vi "IB_RW_Project_Destination_Absolute.vi"(7 "action":T1, 8 "ErrIn":errorcluster, 9 "index":string, 10 "Path":path, 11 "buildObject":T2) -> (0 "ErrOut":errorcluster, 1 "index out":string, 2 "Path":path, 3 "buildObject out":T2)   [LabVIEW 2020]
uses:
  <resource>/Framework/Providers/API/ItemRef.ctl
  <vilib>/AppBuilder/IB_RW_Project/IB_RW_Project_PropBag_Action.ctl
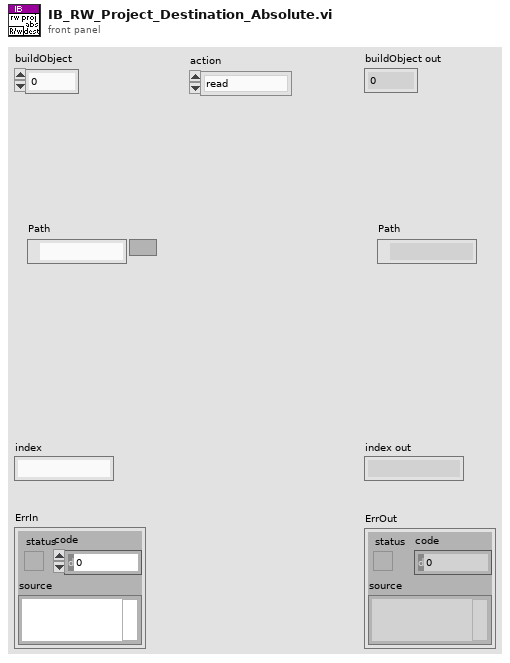
[diagram p1: front panel]
types:
  T1 = typedef "IB_RW_Project_PropBag_Action.ctl" = enum16{"read", "write", "clear", "readPrevious", "writePrevious", "clearPrevious"}
  T2 = typedef "ItemRef.ctl" = u64
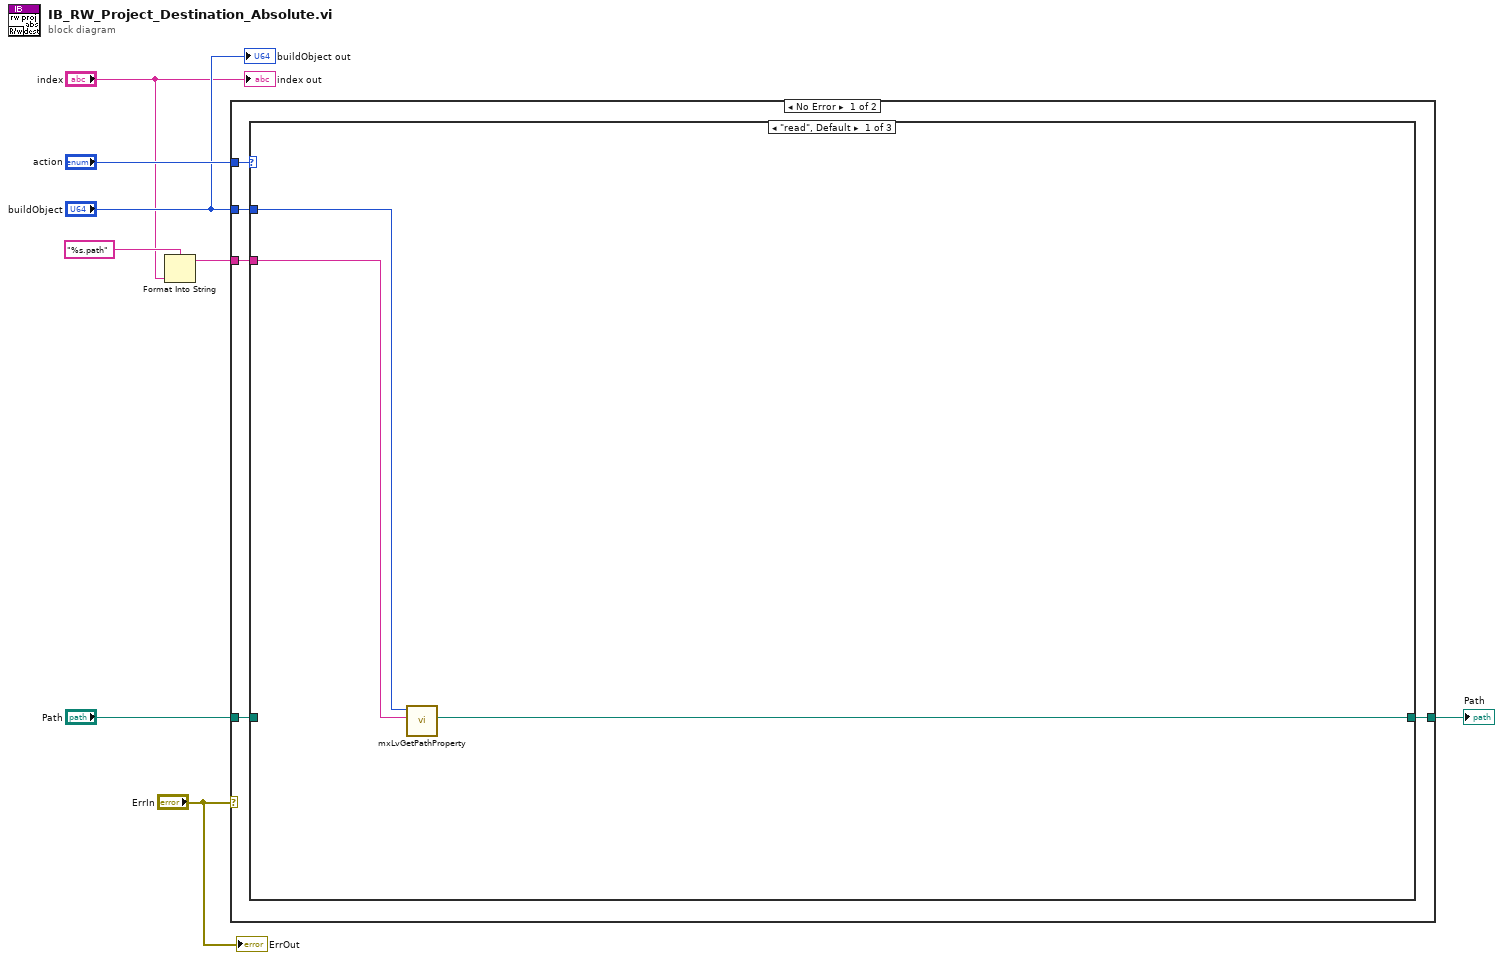
[diagram p0: block diagram]
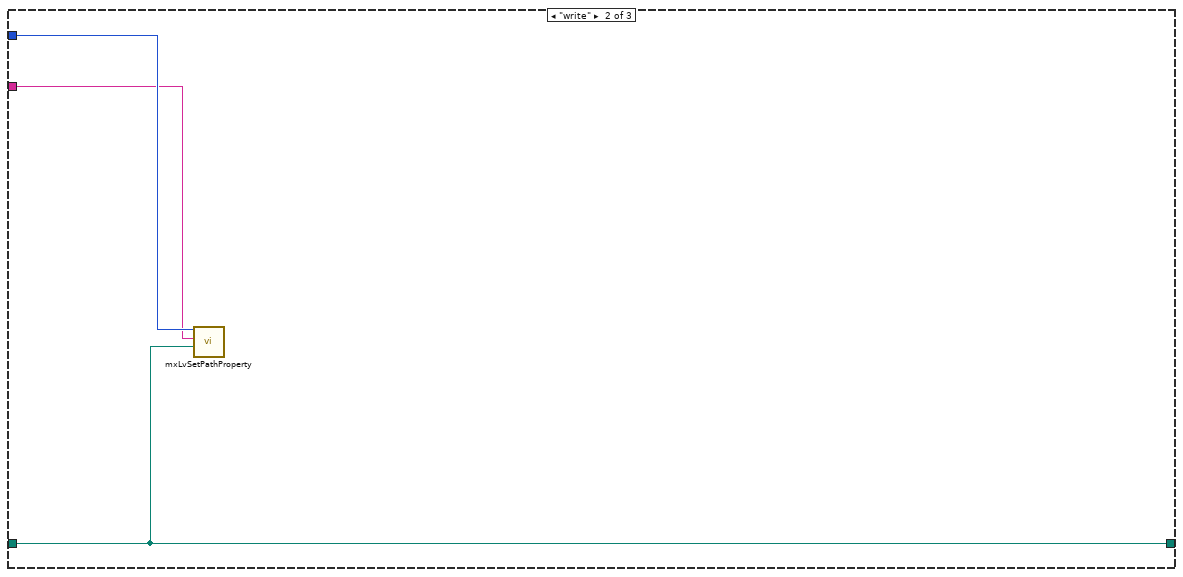
[diagram p2: hidden frame]
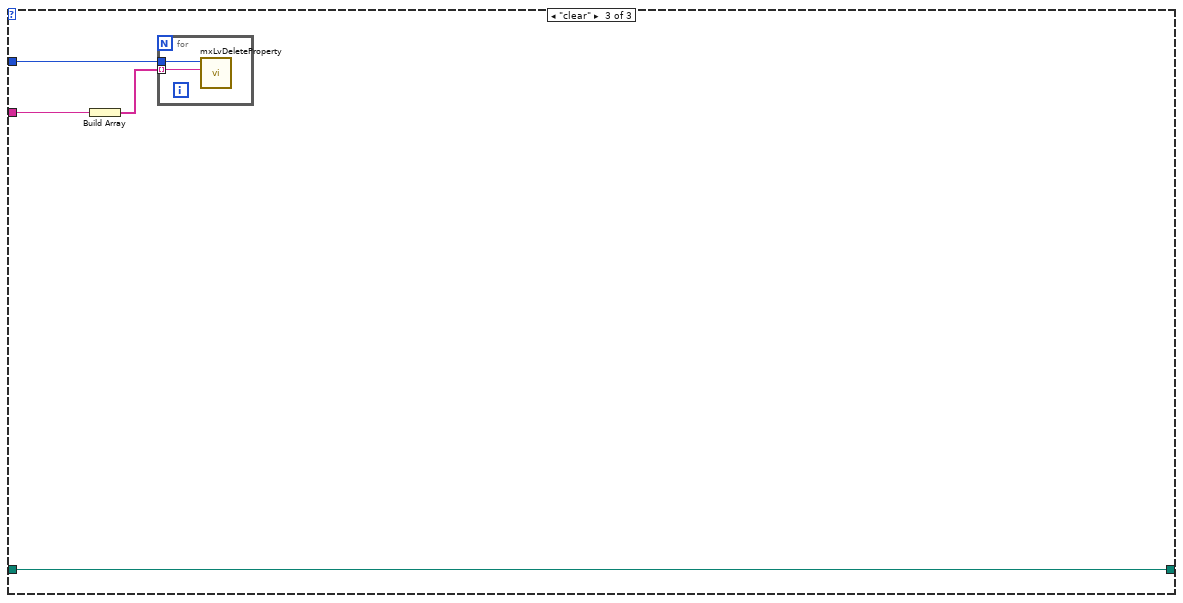
[diagram p3: hidden frame]
diagram:
  n1 = Format Into String(format string="%s.path", "index") -> (resulting string=w4:string)  [unwired: 2 in, 1 out]
  n2 = case shown="No Error" "ErrIn" {
    tunnel: "action" -> [w13 _]
    tunnel: "buildObject" -> [w12 _]
    tunnel: "Path" -> [w11 w26]
    tunnel: [w10 w26] -> w3
    tunnel: w4 -> [w9 _]
    frame No Error {
      n3 = case shown="\"read\", Default" w13 {
        tunnel: w12 -> [w16 w19 w23]
        tunnel: w11 -> [_ w17 w20]
        tunnel: [w14 w17 w20] -> w10
        tunnel: w9 -> [w15 w18 w22]
        frame "read", Default {
          n4 = call <resource>:"mxLvGetPathProperty.vi"("Tag"=w15, "Item"=w16) -> ("Path"=w14:path)  [unwired: 7 in, 2 out]
        }
        frame "write" {
          n5 = call <resource>:"mxLvSetPathProperty.vi"("Path"=w17, "Tag"=w18, "Item"=w19) -> ()  [unwired: 7 in, 2 out]
        }
        frame "clear" {
          n6 = Build Array(w22) -> (w21:string[])
          n7 = for {
            tunnel: w23 -> [w25]
            tunnel: w21 -> [w24] mode=indexing
            n8 = call <resource>:"mxLvDeleteProperty.vi"("Tag"=w24, "Item"=w25) -> ()  [unwired: 1 in, 9 out]
          }
        }
      }
    }
    frame Error {
    }
  }
  "Path" <- w3
  "buildObject out" <- "buildObject"
  "ErrOut" <- "ErrIn"
  "index out" <- "index"
